vi "parse_analog_output_state.vi"(4 "error in":errorcluster, 7 "msg in":string) -> (0 "error out":errorcluster, 2 "Analog State":cluster{"Name":string, "Value":u16}, 3 "msg out":string)   [LabVIEW 2015]
doc: "Parses a message into an analog output"
uses:
  std_msgs/subs/parse_string_scalar.vi
  std_msgs/subs/parse_u16_scalar.vi
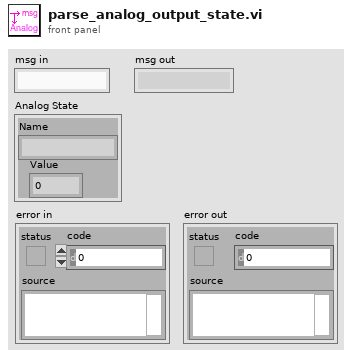
[diagram p1: front panel]
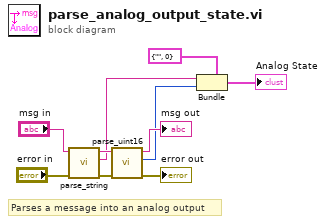
[diagram p0: block diagram]
diagram:
  # "Parses a message into an analog output"
  n1 = call-poly "parse_string.vi"("error in"="error in", "msg in"="msg in") -> ("error out"=w9:errorcluster, "string"=w3:string, "msg out"=w8:string)  [unwired: 3 in]
  n2 = call-poly "parse_uint16.vi"("error in"=w9, "msg in"=w8) -> ("error out"=→"error out":errorcluster, "number"=w2:u16, "msg out"=→"msg out":string)  [unwired: 3 in]
  n3 = Bundle(cluster=cluster{string, i32} {"", 0}, w3, w2) -> (→"Analog State":cluster{string, i32})
